vi "Test Format LogRecord.vi"(8 "error in":errorcluster) -> (0 "error out":errorcluster)   [LabVIEW 2016, in "UT_JSONLFormatter.lvlib"]
doc: "Test the processing of a JSONLines LogRecord."
uses:
  UT_JSONLFormatter.lvlib
  Source/HSE-Logger/LogLevel.ctl
  Source/HSE-Logger/LogRecord/LogRecord.lvclass/LogRecord.ctl
  Source/HSE-Logger/Formatter/JSONLFormatter/JSONLFormatter.lvclass
  C:/Users/admin/_Git/hse-logger/Source/HSE-Logger/Formatter/Formatter.lvclass
  Source/HSE-Logger/Handler/FileHandler/FileHandler.lvclass
  <vilib>/addons/_JKI Toolkits/Caraya/classes/Test/Test.lvclass
  Source/HSE-Logger/hse-logger.lvlib
  Source/HSE-Logger/LogRecord/LogRecord.lvclass
  <vilib>/addons/_JKI Toolkits/Caraya/classes/Assert/Assert.lvclass
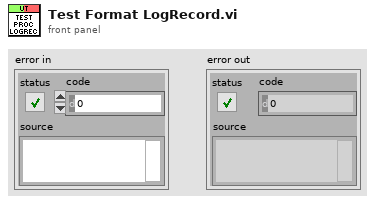
[diagram p1: front panel]
types:
  T1 = typedef "hse-logger.lvlib/LogLevel.ctl" = enum16{"DEBUG", "INFO", "WARNING", "ERROR", "CRITICAL"}
  T2 = enum16{"open", "replace", "create", "open or create", "replace or create", "replace or create with confirmation"}
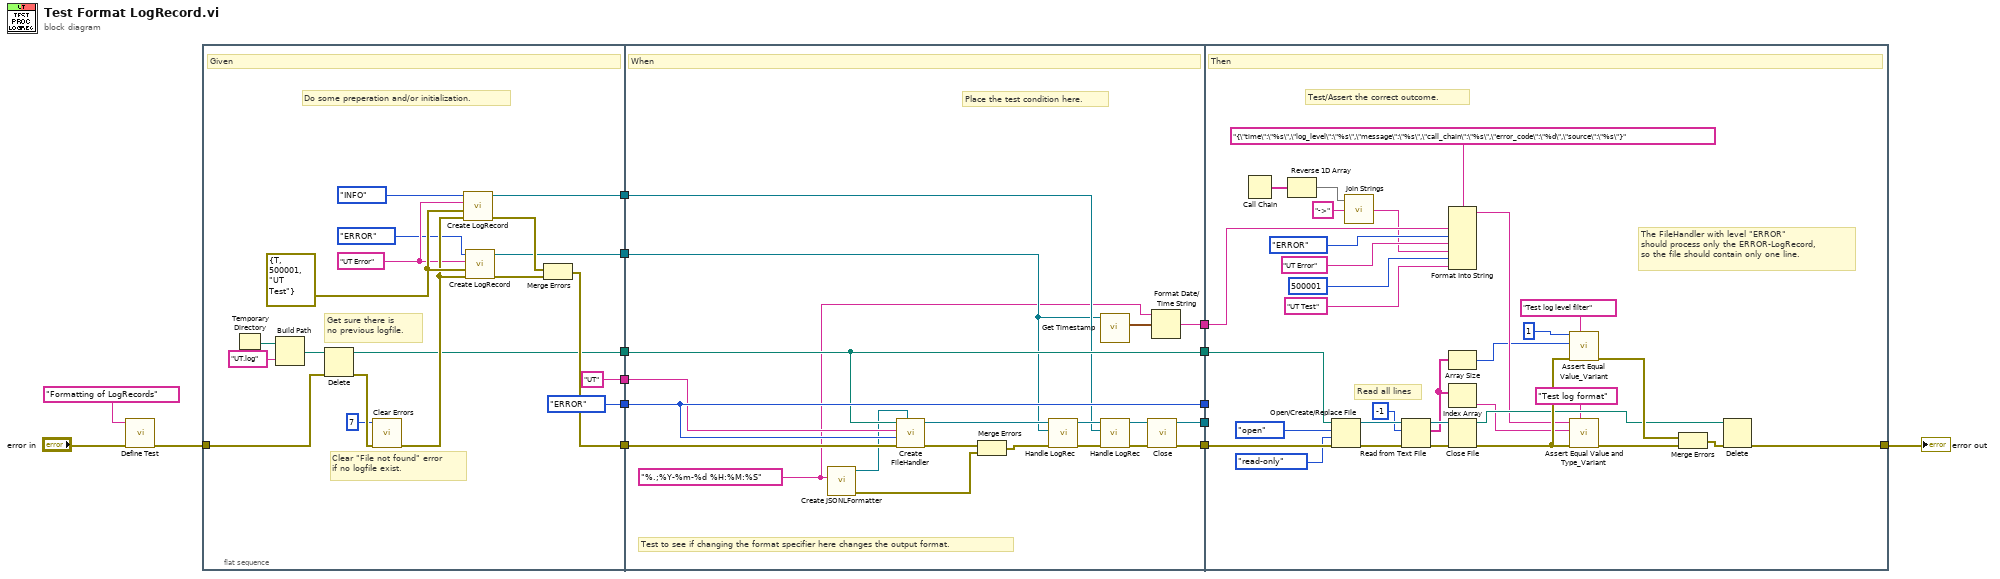
[diagram p0: block diagram]
diagram:
  n1 = call <vilib>:"Define Test.vi"("error in (no error)"="error in", "Label (VI Title)"="Formatting of LogRecords") -> ("error out"=w12:errorcluster)  [unwired: 8 in, 1 out]
  n2 = flat-sequence {
    tunnel: w12 -> [w34]
    tunnel: [w29] -> w15
    tunnel: [LogLevel."ERROR" ("Level")] -> w9
    tunnel: ["UT" ("Name")] -> w8
    tunnel: [w22] -> w7
    tunnel: [w20] -> w3
    tunnel: [w18] -> w2
    tunnel: w15 -> [w54]
    tunnel: [w53] -> w11
    tunnel: w9 -> [w47]
    tunnel: w8 -> [w46]
    tunnel: w7 -> [w45]
    tunnel: [w44] -> w6
    tunnel: [w47] -> w5
    tunnel: [w45] -> w4
    tunnel: w3 -> [w39]
    tunnel: w2 -> [w41]
    tunnel: [w36] -> w1
    tunnel: [w80] -> w14
    tunnel: w11 -> [w85]
    tunnel: w6 -> [_]
    tunnel: w5 -> [_]
    tunnel: w4 -> [w78]
    tunnel: w1 -> [w63]
    frame #0 {
      w31 = errorcluster {"status"=TRUE, "code"=500001, "source"="UT Test"} ("Error to Log")
      w19 = "UT Error" ("Message")
      # "Clear \"File not found\" error\nif no logfile exist."
      # "Get sure there is\nno previous logfile."
      # "Do some preperation and/or initialization."
      # "Given"
      n3 = Temporary Directory() -> (w25:path)
      n4 = Build Path(base path=w25, name or relative path="UT.log") -> (appended path=w23:path)
      n5 = Delete(path (use dialog)=w23, error in=w34) -> (deleted path=w22:path, error out=w33:errorcluster)  [unwired: 3 in, 1 out]
      n6 = call <vilib>:"Clear Errors.vi"("error in (no error)"=w33, "specific error code to clear (0: all)"=7) -> ("error out"=w30:errorcluster)  [unwired: 4 in, 1 out]
      n7 = call "Create LogRecord.vi"("error in"=w30, "Error to Log"=w31, "Message"=w19, "Level"=LogLevel."INFO") -> ("error out"=w28:errorcluster, "LogRecord out"=w18:refnum<class "LogRecord.lvclass">)  [unwired: 6 in]
      n8 = call "Create LogRecord.vi"("error in"=w30, "Error to Log"=w31, "Message"=w19, "Level"=LogLevel."ERROR") -> ("error out"=w32:errorcluster, "LogRecord out"=w20:refnum<class "LogRecord.lvclass">)  [unwired: 6 in]
      n9 = Merge Errors(w28, w32) -> (w29:errorcluster)
    }
    frame #1 {
      w37 = "%.;%Y-%m-%d %H:%M:%S" ("Datetime format")
      # "Test to see if changing the format specifier here changes the output format."
      # "Place the test condition here."
      # "When"
      n10 = call "Create JSONLFormatter.vi"("Datetime format"=w37) -> ("error out"=w49:errorcluster, "JSONLFormatter out"=w35:refnum<class "JSONLFormatter.lvclass">)  [unwired: 9 in]
      n11 = call "Create FileHandler.vi"("Formatter.lvclass"=w35, "error in"=w54, "Level"=w47, "Name"=w46, "Filepath"=w45) -> ("error out"=w48:errorcluster, "FileHandler out"=w40:refnum<class "FileHandler.lvclass">)  [unwired: 5 in]
      n12 = Merge Errors(w48, w49) -> (w50:errorcluster)
      n13 = call-dynamic "Handle LogRec.vi"("error in"=w50, "LogRecord"=w39, "FileHandler in"=w40) -> ("error out"=w52:errorcluster, "FileHandler out"=w43:refnum<class "FileHandler.lvclass">)  [unwired: 7 in]
      n14 = call "Get Timestamp.vi"("LogRecord in"=w39) -> ("Created"=w38:timestamp)  [unwired: 8 in, 2 out]
      n15 = call-dynamic "Handle LogRec.vi"("error in"=w52, "LogRecord"=w41, "FileHandler in"=w43) -> ("error out"=w51:errorcluster, "FileHandler out"=w42:refnum<class "FileHandler.lvclass">)  [unwired: 7 in]
      n16 = call-dynamic "Close.vi"("error in"=w51, "FileHandler in"=w42) -> ("error out"=w53:errorcluster, "FileHandler out"=w44:refnum<class "FileHandler.lvclass">)  [unwired: 8 in]
      n17 = Format Date/Time String(time format string (%c)=w37, seconds (now)=w38) -> (date/time string=w36:string)  [unwired: 1 in]
    }
    frame #2 {
      # "The FileHandler with level \"ERROR\"\nshould process only the ERROR-LogRecord,\nso the file should contain only one line."
      # "Read all lines"
      # "Test/Assert the correct outcome."
      # "Then"
      n18 = Call Chain() -> (call chain=w56:string[])
      n19 = Reverse 1D Array(array=w56) -> (reversed array=w55:string[])
      n20 = Open/Create/Replace File(file path (use dialog)=w78, error in=w85, operation (0:open)=T2."open", access (0:read/write)=enum16{"read/write", "read-only", "write-only"}."read-only") -> (refnum out=w75:refnum<file>, error out=w84:errorcluster)  [unwired: 2 in, 1 out]
      n21 = call <vilib>:"Join Strings.vi"("Separator (,)"="->", "Strings In"=w55) -> ("String"=w60:string)  [unwired: 1 in]
      n22 = Read from Text File(file (use dialog)=w75, count=-1, error in=w84) -> (refnum out=w74:refnum<file>, text=w69:string[], error out=w82:errorcluster)  [unwired: 1 in, 1 out]
      n23 = Format Into String(format string="{\"time\":\"%s\",\"log_level\":\"%s\",\"message\":\"%s\",\"call_chain\":\"%s\",\"error_code\":\"%d\",\"source\":\"%s\"}", w63, LogLevel."ERROR" ("Level"), "UT Error" ("Message"), w60, 500001 ("code"), "UT Test" ("Message")) -> (resulting string=w72:string)  [unwired: 2 in, 1 out]
      n24 = Array Size(array=w69) -> (size(s)=w67:i32)
      n25 = Index Array(array=w69) -> (element=w70:string)  [unwired: 1 in]
      n26 = Close File(refnum=w74, error in=w82) -> (path=w73:path, error out=w79:errorcluster)
      n27 = call <vilib>:"Assert Equal Value_Variant.vi"("Label"="Test log level filter", "error in (no error)"=w79, "Y"=w67, "X"=1 ("size(s)")) -> ("error out"=w86:errorcluster)  [unwired: 6 in, 1 out]
      n28 = call <vilib>:"Assert Equal Value and Type_Variant.vi"("Label"="Test log format", "error in (no error)"=w79, "Y"=w70, "X"=w72) -> ("error out"=w83:errorcluster)  [unwired: 6 in, 1 out]
      n29 = Merge Errors(w86, w83) -> (w81:errorcluster)
      n30 = Delete(path (use dialog)=w73, error in=w81) -> (error out=w80:errorcluster)  [unwired: 3 in, 2 out]
    }
  }
  "error out" <- w14
